vi "BfrPkt - Set Buffer Direction.vi"(8 "error in (no error)":errorcluster, 10 "External?":bool, 11 "Node Ptr":T1 format="%.0x") -> (0 "error out":errorcluster, 3 "Node Ptr out":T1 format="%.0x")   [LabVIEW 2016, in "UDP-Custom-Device System Explorer.lvlib"]
uses:
  UDP-Custom-Device System Explorer.lvlib
  <vilib>/NI Veristand/Custom Device API/Custom Device Item Ref.ctl
  <vilib>/NI Veristand/Custom Device API/Custom Device Channel Type.ctl
  <vilib>/NI VeriStand/Custom Device API/Custom Device API.lvlib
  <vilib>/NI VeriStand/Custom Device Tools/Custom Device Utility Library/Custom Device Utility Library.lvlib
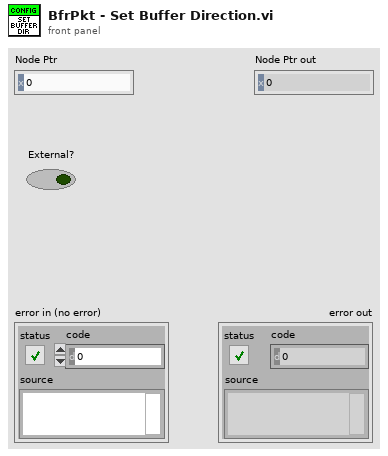
[diagram p1: front panel]
types:
  T1 = typedef "Custom Device API.lvlib/Custom Device Item Ref.ctl" = u64
  T2 = typedef "Custom Device API.lvlib/Custom Device Channel Type.ctl" = enum16{"Input", "Output"}
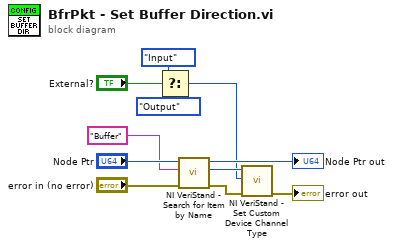
[diagram p0: block diagram]
diagram:
  n1 = Select(t=Custom_Device_Channel_Type."Input" ("Type"), s="External?", f=Custom_Device_Channel_Type."Output" ("Type")) -> (s? t:f=w1:T2)
  n2 = call <vilib>:"NI VeriStand - Search for Item by Name.vi"("error in"="error in (no error)", "Item Name"="Buffer", "Section Ref in"="Node Ptr") -> ("error out"=w9:errorcluster, "Item Ref"=w6:T1, "Section Ref out"=→"Node Ptr out":T1)  [unwired: 5 in, 1 out]
  n3 = call <vilib>:"NI VeriStand - Set Custom Device Channel Type.vi"("error in (no error)"=w9, "Type"=w1, "Channel Ref in"=w6) -> ("error out"=→"error out":errorcluster)  [unwired: 7 in, 1 out]
